vi "Subvi Calculate Exposure Type.vi"(1 "CutsCompleted":u32) -> (0 "ThisPass":u16(ring) items=["Brightfield", "Fluorescence", "Both"])   [LabVIEW 2012]
uses:
  ProSCI Global.vi
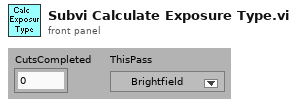
[diagram p1: front panel]
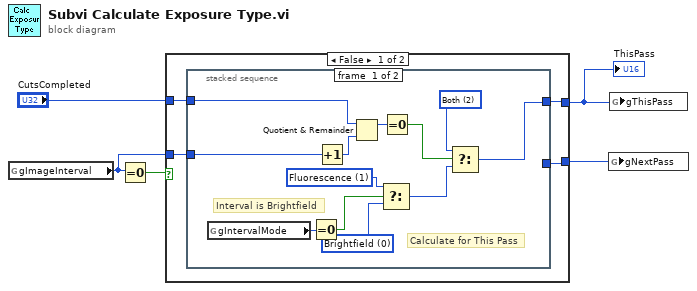
[diagram p0: block diagram]
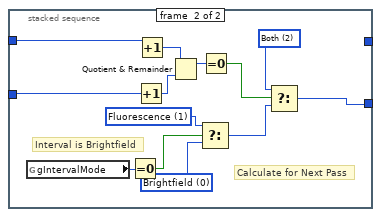
[diagram p2: hidden frame]
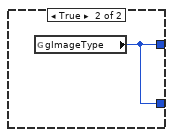
[diagram p3: hidden frame]
diagram:
  n1 = global read "ProSCI Global.vi" "gImageInterval"() -> (w3:i32)
  n2 = Equal To 0?(x=w3) -> (x = 0?=w5:bool)
  n3 = case shown="False" w5 {
    tunnel: [w8 w35] -> w2
    tunnel: [w7 w35] -> w4
    tunnel: w3 -> [w9 _]
    tunnel: "CutsCompleted" -> [w6 _]
    frame False {
      n4 = stacked-sequence {
        tunnel: w9 -> [w19 w25]
        tunnel: [w16 _] -> w8
        tunnel: [_ w24] -> w7
        tunnel: w6 -> [w10 w22]
        frame #0 {
          w12 = u16 0 items=["Brightfield", "Fluorescence", "Both"] ("gThisPass")
          w13 = u16 1 items=["Brightfield", "Fluorescence", "Both"] ("gThisPass")
          w17 = u16 2 items=["Brightfield", "Fluorescence", "Both"] ("gThisPass")
          # "Calculate for This Pass"
          # "Interval is Brightfield"
          n5 = global read "ProSCI Global.vi" "gIntervalMode"() -> (w15:i8)
          n6 = Equal To 0?(x=w15) -> (x = 0?=w14:bool)
          n7 = Increment(x=w19) -> (x+1=w21:i32)
          n8 = Quotient & Remainder(x=w10, y=w21) -> (x-y*floor(x/y)=w20:u32)  [unwired: 1 out]
          n9 = Select(t=w13, s=w14, f=w12) -> (s? t:f=w11:u16)
          n10 = Equal To 0?(x=w20) -> (x = 0?=w18:bool)
          n11 = Select(t=w17, s=w18, f=w11) -> (s? t:f=w16:u16)
        }
        frame #1 {
          w33 = u16 0 items=["Brightfield", "Fluorescence", "Both"] ("gThisPass")
          w32 = u16 1 items=["Brightfield", "Fluorescence", "Both"] ("gThisPass")
          w29 = u16 2 items=["Brightfield", "Fluorescence", "Both"] ("gThisPass")
          # "Calculate for Next Pass"
          # "Interval is Brightfield"
          n12 = global read "ProSCI Global.vi" "gIntervalMode"() -> (w30:i8)
          n13 = Equal To 0?(x=w30) -> (x = 0?=w31:bool)
          n14 = Increment(x=w25) -> (x+1=w26:i32)
          n15 = Increment(x=w22) -> (x+1=w23:u32)
          n16 = Quotient & Remainder(x=w23, y=w26) -> (x-y*floor(x/y)=w27:u32)  [unwired: 1 out]
          n17 = Select(t=w32, s=w31, f=w33) -> (s? t:f=w34:u16)
          n18 = Equal To 0?(x=w27) -> (x = 0?=w28:bool)
          n19 = Select(t=w29, s=w28, f=w34) -> (s? t:f=w24:u16)
        }
      }
    }
    frame True {
      n20 = global read "ProSCI Global.vi" "gImageType"() -> (w35:i8)
    }
  }
  "ThisPass" <- w2
  n21 = global write "ProSCI Global.vi" "gNextPass"(w4) -> ()
  n22 = global write "ProSCI Global.vi" "gThisPass"(w2) -> ()
